vi "Module Not Running--error.vi"() -> (0 "error out":errorcluster)   [LabVIEW 2020, in "Money.lvlib"]
doc: "Outputs an error cluster containing a custom error code indicating the module is not running.\n_____\nBased on Delacor QMH Project Template 4.2.1.64."
uses:
  Money.lvlib
  <vilib>/Utility/error.llb/Error Cluster From Error Code.vi
  <vilib>/ErrorRing/Error Ring.xnode
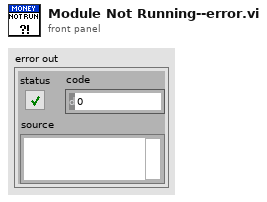
[diagram p1: front panel]
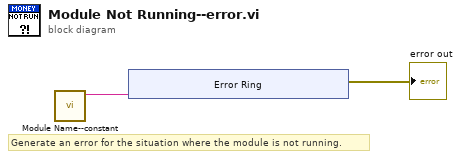
[diagram p0: block diagram]
diagram:
  # "Generate an error for the situation where the module is not running."
  n1 = call "Module Name--constant.vi"() -> ("Module Name"=w1:string)  [unwired: 11 in]
  n2 = xnode "Error Ring"("parameter 0"=w1) -> ("error out"=→"error out":errorcluster)
